vi "IV_analysis_tdms_IV_ranjani.vi"() -> ()   [LabVIEW 2020]
uses:
  <userlib>/LevyLab/LV-Data/LV-Data.ITX/Typedefs/Retrieve Data Type.ctl
  <userlib>/LevyLab/LV-Data/LV-Data.ITX/LV-Data.ITX.lvclass
panel:
  in  "fake point value":dbl=-1.0 format="%#_6p"
  out "IV":cluster{dbl[], dbl[]}[](graph)
  out "Conductance":cluster{dbl[], dbl[]}[](graph)
  in  "average length":i32=100
  in  "dv":dbl=15.0 format="%#_13g"
  out "?":dbl[][](graph)
  out "?":dbl[][](graph)
  out "?":dbl[][](graph)
  in  "X Step":dbl=1e-05 format="%#_6p"
  in  "X High":dbl=0.012 format="%#_6p"
  in  "X Low":dbl=-0.012 format="%#_6p"
  in  "# per group":i32=1
  in  "Group #":i32=28
  in  "File or Folder Path 2":path=path "G:/.shortcut-targets-by-id/0B8-gGFa6hkR4XzJJMDlqZXVKRk0/ansom/Data/PPMSDAQ/2022/PPMS 1/SA40286I.20220426/15-Tsweep_20V"
  in  "LV to itx":T1={"A"=10, "B"=5, "C"=4, "D"=0, "E"=0, "N1"=5, "N2"=0, "N3"=0, "N4"=0}
  in  "index in group":i32
  in  "File_index":i32
  in  "offset":i32=1
  in  "LV/ITX?":bool=TRUE
  # "Current"
  # "V4T+"
  # "10/5 4 for Tsweep"
  # "V4T-"
  # "11/6 5 for Bsweep/Vbgsweep"
  # "Drive current"
  # "Vbg/Vsg"
  # "Temp/B"
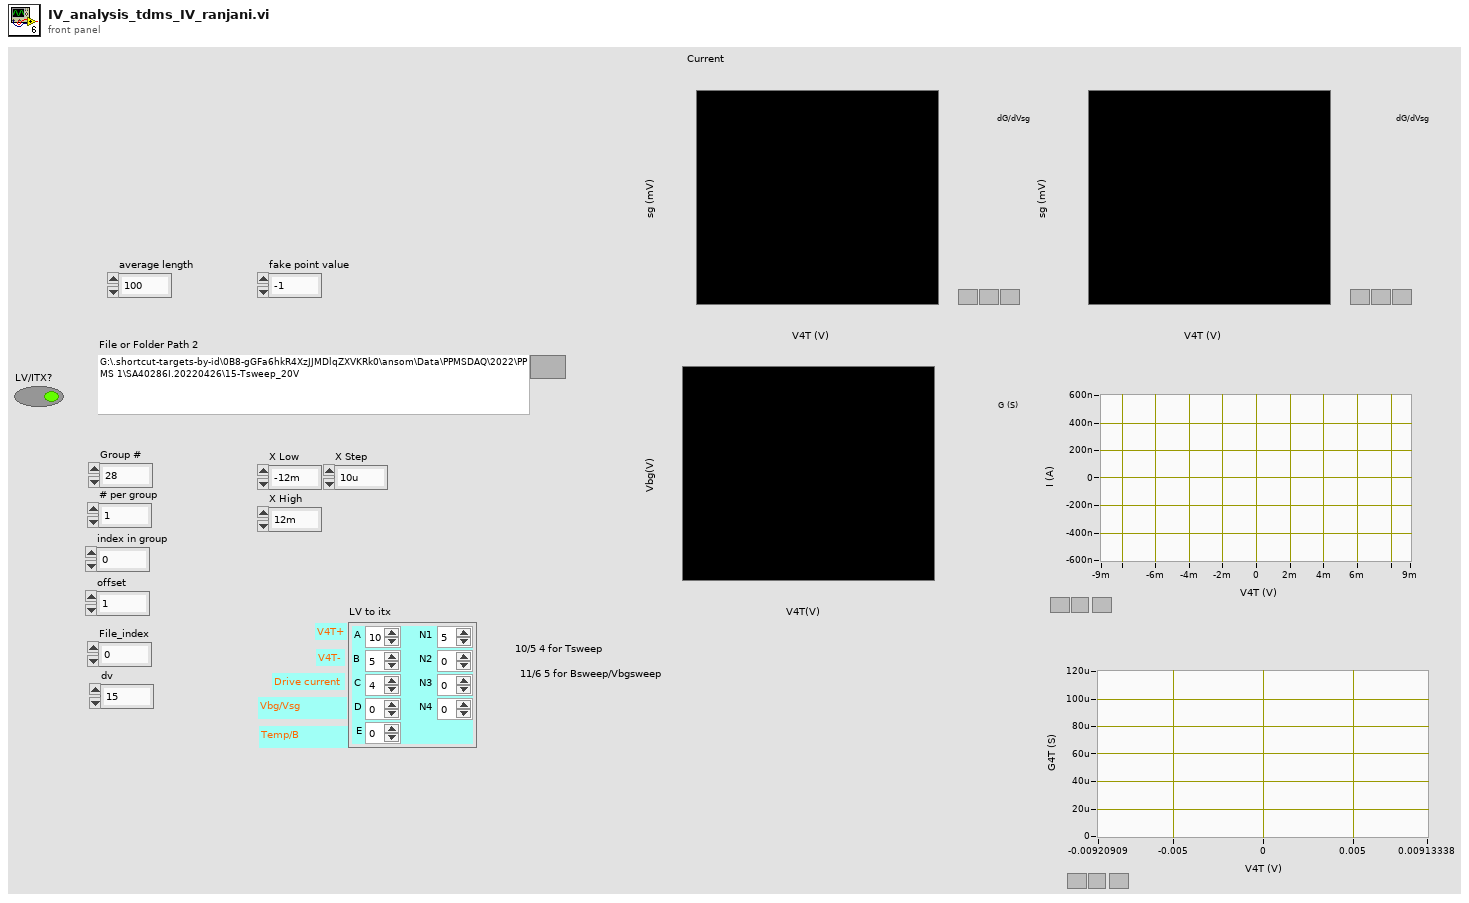
[diagram p1: front panel]
types:
  T1 = cluster{"A":i32, "B":i32, "C":i32, "D":i32, "E":i32, "N1":i32, "N2":i32, "N3":i32, "N4":i32}
  T2 = typedef "LV-Data.ITX.lvclass/Retrieve Data Type.ctl" = enum16{"ITX", "ITX w/ 2D", "DAT", "TDMS"}
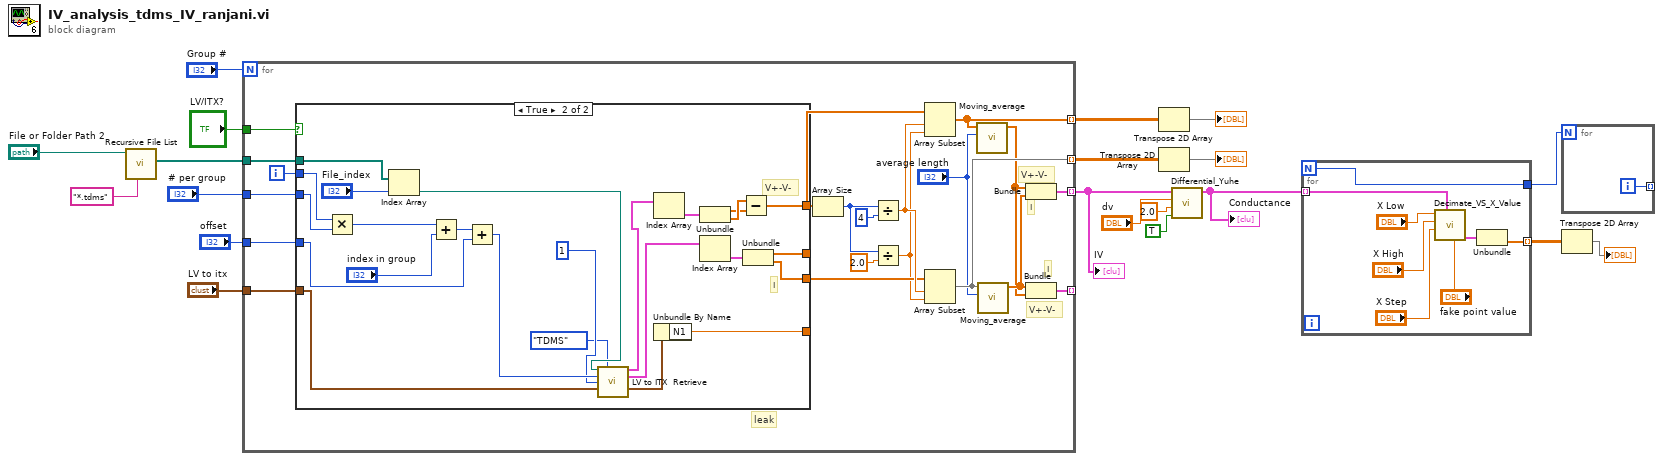
[diagram p0: block diagram]
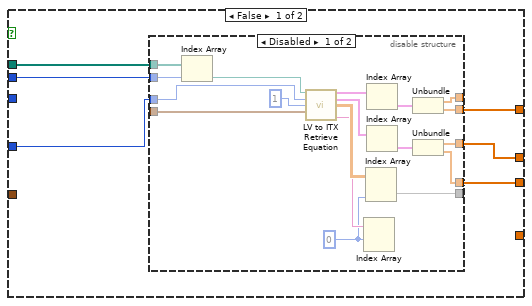
[diagram p2: hidden frame]
diagram:
  n1 = call <vilib>:"Recursive File List.vi"("pattern"="*.tdms", "Folder Path"="File or Folder Path 2") -> ("All Files in Dir"=w17:path[])  [unwired: 5 in, 4 out]
  n2 = for {
    N: "Group #" -> [_]
    tunnel: w17 -> [w40]
    tunnel: "LV to itx" -> [w39]
    tunnel: "offset" -> [w38]
    tunnel: "LV/ITX?" -> [w37]
    tunnel: "# per group" -> [w35]
    tunnel: [w34] -> w2 mode=indexing
    tunnel: [w26] -> w7 mode=indexing
    tunnel: [w25] -> w5 mode=indexing
    tunnel: [w21] -> _ mode=indexing
    i -> [w36]
    # "V+-V-"
    # "I"
    # "I"
    # "V+-V-"
    # "leak"
    n3 = case shown="True" w37 {
      tunnel: w40 -> [w42 w88]
      tunnel: w39 -> [_ w73]
      tunnel: [w45 w79] -> _
      tunnel: [w44 w80] -> w28
      tunnel: [_ w89] -> _
      tunnel: [w46 w74] -> w29
      tunnel: w38 -> [w43 w87]
      tunnel: w36 -> [w41 w86]
      tunnel: w35 -> [_ w85]
      frame False {
        n4 = disable-structure shown="Disabled" {
          disable-tunnel: _ -> [w65 _]
          disable-tunnel: [w58 _] -> _
          disable-tunnel: [w57 _] -> w46
          disable-tunnel: [w56 _] -> w45
          disable-tunnel: [w55 _] -> w44
          disable-tunnel: [w54 _] -> _
          disable-tunnel: w43 -> [w53 _]
          disable-tunnel: w42 -> [w49 _]
          disable-tunnel: w41 -> [w48 _]
          frame Disabled {
            w50 = 0 ("length")
            n5 = Index Array(array=w49, index=w48) -> (element=w47:path)
            n6 = call <userlib>:"LV to ITX  Retrieve Equation.vi"("File or Folder Path"=w47, "offset"=w53, "length"=1, "index"=w65) -> ("y1 vs g"=w63:cluster{dbl[], dbl[]}[], "y2 vs g"=w61:cluster{dbl[], dbl[]}[], "2D"=w59:dbl[][], "Comments"=w52:string)  [unwired: 7 in, 1 out]
            n7 = Index Array(array=w52, index (row)=w50) -> (element=w51)  [unwired: 1 in]
            n8 = Index Array(array=w59, index (col)=w50) -> (element=w54:dbl[])  [unwired: 1 in]
            n9 = Index Array(array=w63) -> (element=w62:cluster{dbl[], dbl[]})  [unwired: 1 in]
            n10 = Index Array(array=w61) -> (element=w60:cluster{dbl[], dbl[]})  [unwired: 1 in]
            n11 = Unbundle(w62) -> (w58:dbl[], w57:dbl[])
            n12 = Unbundle(w60) -> (w56:dbl[], w55:dbl[])
          }
          frame Enabled {
          }
        }
      }
      frame True {
        # "I"
        # "V+-V-"
        n13 = Multiply(x=w86, y=w85) -> (x*y=w84:i32)
        n14 = Index Array(array=w88, index="File_index") -> (element=w71:path)
        n15 = Add(x=w84, y="index in group") -> (x+y=w82:i32)
        n16 = Add(x=w82, y=w87) -> (x+y=w70:i32)
        n17 = call <userlib>:"LV to ITX  Retrieve.vi"("File or Folder Path"=w71, "Data Type"=Retrieve_Data_Type."TDMS", "offset"=w70, "length"=1, "index"=w73) -> ("A vs B"=w67:cluster{dbl[], dbl[]}[], "C vs D"=w68:cluster{dbl[], dbl[]}[], "N"=w72:cluster{"N1":dbl, "N2":dbl, "N3":dbl, "N4":dbl})  [unwired: 5 in, 3 out]
        n18 = Index Array(array=w67) -> (element=w78:cluster{dbl[], dbl[]})  [unwired: 1 in]
        n19 = Unbundle By Name(w72) -> ("N1"=w89:dbl)
        n20 = Unbundle(w78) -> (w76:dbl[], w77:dbl[])
        n21 = Index Array(array=w68) -> (element=w81:cluster{dbl[], dbl[]})  [unwired: 1 in]
        n22 = Subtract(x=w77, y=w76) -> (x-y=w74:dbl[])
        n23 = Unbundle(w81) -> (w79:dbl[], w80:dbl[])
      }
    }
    n24 = Array Size(array=w29) -> (size(s)=w31:i32)
    n25 = Divide(x=w31, y=4) -> (x/y=w30:dbl)
    n26 = Divide(x=w31, y=2.0) -> (x/y=w27:dbl)
    n27 = Array Subset(array=w29, index=w30, length=w27) -> (w25:dbl[])
    n28 = Array Subset(array=w28, index=w30, length=w27) -> (w26:dbl[])
    n29 = call "Moving_average.vi"("average length"="average length", "Input"=w25) -> ("Output"=w22:dbl[])  [unwired: 9 in]
    n30 = call "Moving_average.vi"("average length"="average length", "Input"=w26) -> ("Output"=w23:dbl[])  [unwired: 9 in]
    n31 = Bundle("Output"=w22, "Output"=w23) -> (w34:cluster{"Output":dbl[], "Output":dbl[]})  [unwired: 1 in]
    n32 = Bundle("Output"=w23, "Output"=w22) -> (w21:cluster{"Output":dbl[], "Output":dbl[]})  [unwired: 1 in]
  }
  "IV" <- w2
  n33 = Transpose 2D Array(2D array=w5) -> (transposed array=→"?":dbl[][])
  n34 = Transpose 2D Array(2D array=w7) -> (transposed array=→"?":dbl[][])
  n35 = call "Differential_Yuhe.vi"("dy/dx vs x"=TRUE, "step"=2.0, "dv"="dv", "A vs B"=w2) -> ("A vs B 2"=w3:cluster{dbl[], dbl[]}[])  [unwired: 7 in]
  "Conductance" <- w3
  n36 = for {
    N -> [w91]
    tunnel: w3 -> [w97] mode=indexing
    tunnel: [w92] -> w10 mode=indexing
    tunnel: [w91] -> w9
    n37 = call "Decimate_VS_X_Value.vi"("fake point value"="fake point value", "XY Graph kind 1"=w97, "X Step"="X Step", "X High"="X High", "X Low"="X Low") -> ("Interpreted"=w93:cluster{dbl[], dbl[]})  [unwired: 5 in, 1 out]
    n38 = Unbundle(w93) -> (w92:dbl[])  [unwired: 1 out]
  }
  n39 = for {
    N: w9 -> [_]
    tunnel: [w98] -> _ mode=indexing
    i -> [w98]
  }
  n40 = Transpose 2D Array(2D array=w10) -> (transposed array=→"?":dbl[][])
